vi "ErwKonf_SysLog.vi"(11 "Cluster":T4 {"Lüfter langsam" format="%#_5g"; "Schnell ab:" format="%#_5g"; "FT-IR Kühlung Soll" format="%#_5g"; "FT-IR Kühlung Max" format="%#_5g"; "Stickstoff Befüllzeit" format="%#_5g"; "Befüllintervall" format="%#_5g"; "Kalib.FT-IR" format="%#_5g"; "Offset Ausgang" format="%#_5g"; "Offset FT-IR" format="%#_5g"; "Offset Druck FT-IR" format="%#_5g"; "Dichtheitstest Zeit" format="%#_5g"; "Dichtheitstest Abfall" format="%#_5g"; "Dichtheitstest Umfang" items=["Pumpe / Filter / FT-IR / PNS", "Pumpe / Filter / FT-IR", "Filter / FT-IR", "FT-IR"]; "Offset Umgebung" format="%#_5g"; "Max Taupunkt" format="%#_5g"}) -> (3 "Cluster out":T4 {"Lüfter langsam" format="%#_5g"; "Schnell ab:" format="%#_5g"; "FT-IR Kühlung Soll" format="%#_5g"; "FT-IR Kühlung Max" format="%#_5g"; "Stickstoff Befüllzeit" format="%#_5g"; "Befüllintervall" format="%#_5g"; "Kalib.FT-IR" format="%#_5g"; "Offset Ausgang" format="%#_5g"; "Offset FT-IR" format="%#_5g"; "Offset Druck FT-IR" format="%#_5g"; "Dichtheitstest Zeit" format="%#_5g"; "Dichtheitstest Abfall" format="%#_5g"; "Dichtheitstest Umfang" items=["Pumpe / Filter / FT-IR / PNS", "Pumpe / Filter / FT-IR", "Filter / FT-IR", "FT-IR"]; "Offset Umgebung" format="%#_5g"; "Max Taupunkt" format="%#_5g"})   [LabVIEW 2020, in "Erweiterte Konfig.lvlib"]
uses:
  Erweiterte Konfig.lvlib
  Visualisierungs Elemente/Zahlen-Eingabefeld.ctl
  Visualisierungs Elemente/Auswahlfeld.ctl
  Dichtheitstest Umfang.ctl
  FGV PID Aktionen.ctl
  SysLog/SysLog Interface.ctl
  SysLog/SysLog.lvlib
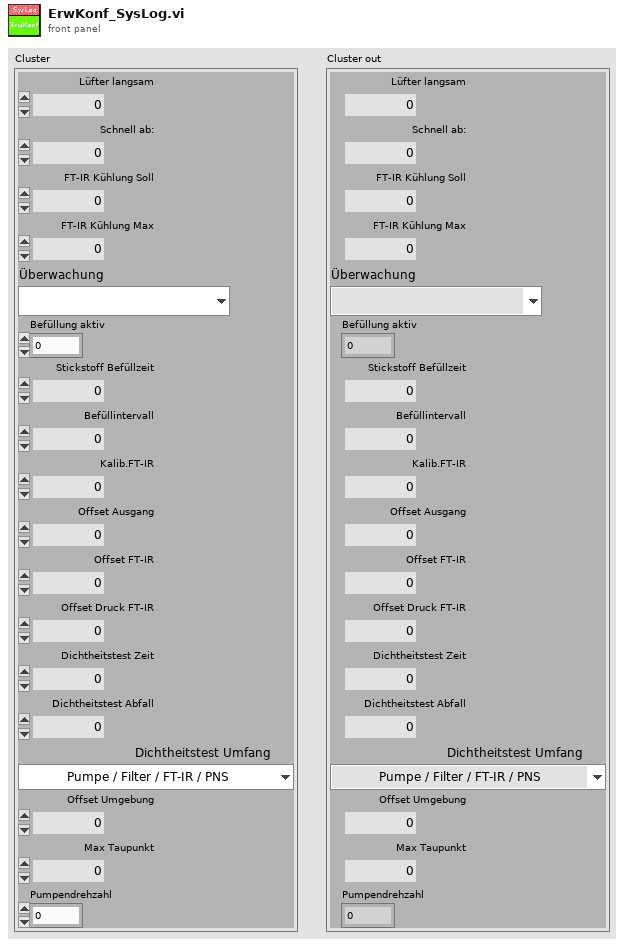
[diagram p1: front panel]
types:
  T1 = typedef "Zahlen-Eingabefeld.ctl" = sgl
  T2 = typedef "Auswahlfeld.ctl" = u16
  T3 = typedef "Erweiterte Konfig.lvlib/Dichtheitstest Umfang.ctl" = u16
  T4 = cluster{"Lüfter langsam":T1, "Schnell ab:":T1, "FT-IR Kühlung Soll":T1, "FT-IR Kühlung Max":T1, "Überwachung":T2, "Befüllung aktiv":u16, "Stickstoff Befüllzeit":T1, "Befüllintervall":T1, "Kalib.FT-IR":T1, "Offset Ausgang":T1, "Offset FT-IR":T1, "Offset Druck FT-IR":T1, "Dichtheitstest Zeit":T1, "Dichtheitstest Abfall":T1, "Dichtheitstest Umfang":T3, "Offset Umgebung":T1, "Max Taupunkt":T1, "Pumpendrehzahl":sgl}
  T5 = typedef "Erweiterte Konfig.lvlib/FGV PID Aktionen.ctl" = enum16{"Lesen", "Schreiben PID", "Schreiben Sonstige", "Dichtheitstest", "Aktionen Dicht.", "Parameter Sensor"}
  T6 = typedef "Erweiterte Konfig.lvlib/Sonstige Parameter.ctl" = cluster{"Lüfter langsam":sgl, "Lüfter schnell":sgl, "FT-IR Kühlung Soll":sgl, "FT-IR Kühlung Max":sgl, "Überwachung":T2, "Befüllung aktiv":T7, "Stickstoff Befüllzeit":sgl, "Befüllintervall":sgl, "Kalibrierwert FT-IR":sgl, "Offset Ausgang":sgl, "Offset FT-IR":sgl, "Offset Druck FT-IR":sgl, "Dichtheitstest Zeit":sgl, "Dichtheitstest Abfall":sgl, "Dichtheitstest Umfang":T3, "Offset Umgebung":sgl, "Max Taupunkt":sgl, "Pumpendrehzahl":sgl}
  T7 = typedef "LogKonfig.lvlib/Auswahlfeld aktiviert-deaktiviert.ctl" = u16
  T8 = typedef "SysLog.lvlib/SysLog Interface.ctl" = cluster{"Fehlermeldung":string, "Erfolgsmeldung":string, "Anzeige":bool, "SysLogIcon":enum16{"OK", "Warnung", "Fehler"}, "intern":bool}
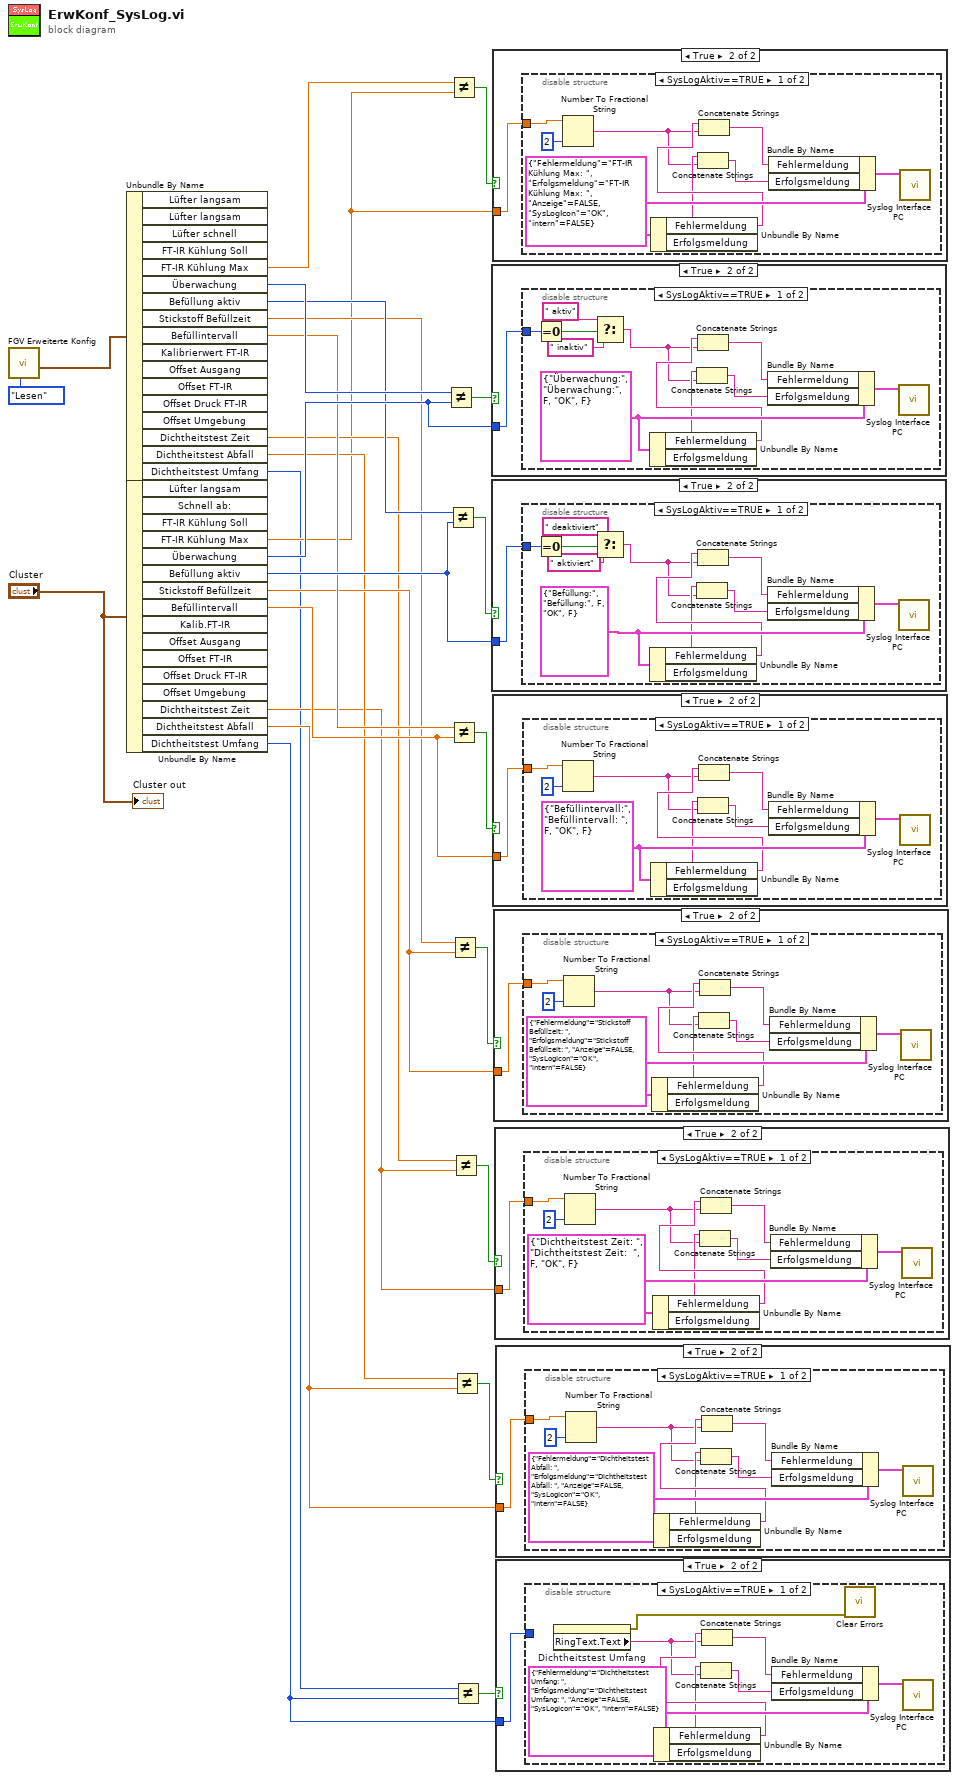
[diagram p0: block diagram]
diagram:
  n1 = call "FGV Erweiterte Konfig.vi"("Aktion"=FGV_PID_Aktionen."Lesen") -> ("Sonstige"=w26:T6)  [unwired: 5 in, 5 out]
  n2 = Unbundle By Name(w26) -> ("FT-IR Kühlung Max"=w5:sgl, "Überwachung"=w24:T2, "Befüllung aktiv"=w21:T7, "Stickstoff Befüllzeit"=w14:sgl, "Befüllintervall"=w17:sgl, "Dichtheitstest Zeit"=w10:sgl, "Dichtheitstest Abfall"=w9:sgl, "Dichtheitstest Umfang"=w3:T3)  [unwired: 9 out]
  n3 = Unbundle By Name("Cluster") -> ("FT-IR Kühlung Max"=w4:T1, "Überwachung"=w22:T2, "Befüllung aktiv"=w19:u16, "Stickstoff Befüllzeit"=w13:T1, "Befüllintervall"=w16:T1, "Dichtheitstest Zeit"=w8:T1, "Dichtheitstest Abfall"=w7:T1, "Dichtheitstest Umfang"=w1:T3)  [unwired: 8 out]
  n4 = Not Equal?(x=w24, y=w22) -> (x != y?=w23:bool)
  n5 = Not Equal?(x=w21, y=w19) -> (x != y?=w20:bool)
  n6 = Not Equal?(x=w5, y=w4) -> (x != y?=w6:bool)
  n7 = Not Equal?(x=w17, y=w16) -> (x != y?=w18:bool)
  n8 = Not Equal?(x=w14, y=w13) -> (x != y?=w15:bool)
  n9 = Not Equal?(x=w10, y=w8) -> (x != y?=w12:bool)
  n10 = Not Equal?(x=w9, y=w7) -> (x != y?=w11:bool)
  n11 = Not Equal?(x=w3, y=w1) -> (x != y?=w2:bool)
  n12 = case shown="True" w23 {
    tunnel: w22 -> [_ w28]
    frame False {
    }
    frame True {
      n13 = disable-structure shown="SysLogAktiv==TRUE" {
        disable-tunnel: w28 -> [w37 _]
        frame condition #0 (active) {
          w39 = T8 {"Fehlermeldung"="Überwachung:", "Erfolgsmeldung"="Überwachung:", "Anzeige"=FALSE, "SysLogIcon"=enum."OK", "intern"=FALSE} ("Cluster (in)")
          n14 = Equal To 0?(x=w37) -> (x = 0?=w38:bool)
          n15 = Select(t=" aktiv", s=w38, f=" inaktiv") -> (s? t:f=w31:string)
          n16 = Unbundle By Name(w39) -> ("Fehlermeldung"=w33:string, "Erfolgsmeldung"=w32:string)
          n17 = Concatenate Strings(w32, w31) -> (w29:string)
          n18 = Concatenate Strings(w33, w31) -> (w30:string)
          n19 = Bundle By Name(cluster=w39, "Fehlermeldung"=w30, "Erfolgsmeldung"=w29) -> (w34:T8)
          n20 = call "Syslog Interface PC.vi"("Cluster (in)"=w34) -> ()  [unwired: 10 in, 1 out]
        }
        frame condition #1 {
        }
      }
    }
  }
  n21 = case shown="True" w20 {
    tunnel: w19 -> [_ w40]
    frame False {
    }
    frame True {
      n22 = disable-structure shown="SysLogAktiv==TRUE" {
        disable-tunnel: w40 -> [w49 _]
        frame condition #0 (active) {
          w51 = T8 {"Fehlermeldung"="Befüllung:", "Erfolgsmeldung"="Befüllung:", "Anzeige"=FALSE, "SysLogIcon"=enum."OK", "intern"=FALSE} ("Cluster (in)")
          n23 = Equal To 0?(x=w49) -> (x = 0?=w50:bool)
          n24 = Select(t=" deaktiviert", s=w50, f=" aktiviert") -> (s? t:f=w43:string)
          n25 = Unbundle By Name(w51) -> ("Fehlermeldung"=w45:string, "Erfolgsmeldung"=w44:string)
          n26 = Concatenate Strings(w44, w43) -> (w41:string)
          n27 = Concatenate Strings(w45, w43) -> (w42:string)
          n28 = Bundle By Name(cluster=w51, "Fehlermeldung"=w42, "Erfolgsmeldung"=w41) -> (w46:T8)
          n29 = call "Syslog Interface PC.vi"("Cluster (in)"=w46) -> ()  [unwired: 10 in, 1 out]
        }
        frame condition #1 {
        }
      }
    }
  }
  n30 = case shown="True" w6 {
    tunnel: w4 -> [_ w52]
    frame False {
    }
    frame True {
      n31 = disable-structure shown="SysLogAktiv==TRUE" {
        disable-tunnel: w52 -> [w55 _]
        frame condition #0 (active) {
          w61 = T8 {"Fehlermeldung"="FT-IR Kühlung Max: ", "Erfolgsmeldung"="FT-IR Kühlung Max: ", "Anzeige"=FALSE, "SysLogIcon"=enum."OK", "intern"=FALSE} ("Cluster (in)")
          n32 = Number To Fractional String(number=w55, precision (6)=i16 2 ("Genauigkeit (6)")) -> (F-format string=w54:string)  [unwired: 2 in]
          n33 = Unbundle By Name(w61) -> ("Fehlermeldung"=w59:string, "Erfolgsmeldung"=w58:string)
          n34 = Concatenate Strings(w58, w54) -> (w56:string)
          n35 = Concatenate Strings(w59, w54) -> (w57:string)
          n36 = Bundle By Name(cluster=w61, "Fehlermeldung"=w57, "Erfolgsmeldung"=w56) -> (w60:T8)
          n37 = call "Syslog Interface PC.vi"("Cluster (in)"=w60) -> ()  [unwired: 10 in, 1 out]
        }
        frame condition #1 {
        }
      }
    }
  }
  n38 = case shown="True" w18 {
    tunnel: w16 -> [_ w62]
    frame False {
    }
    frame True {
      n39 = disable-structure shown="SysLogAktiv==TRUE" {
        disable-tunnel: w62 -> [w65 _]
        frame condition #0 (active) {
          w71 = T8 {"Fehlermeldung"="Befüllintervall:", "Erfolgsmeldung"="Befüllintervall: ", "Anzeige"=FALSE, "SysLogIcon"=enum."OK", "intern"=FALSE} ("Cluster (in)")
          n40 = Number To Fractional String(number=w65, precision (6)=i16 2 ("Genauigkeit (6)")) -> (F-format string=w64:string)  [unwired: 2 in]
          n41 = Unbundle By Name(w71) -> ("Fehlermeldung"=w69:string, "Erfolgsmeldung"=w68:string)
          n42 = Concatenate Strings(w68, w64) -> (w66:string)
          n43 = Concatenate Strings(w69, w64) -> (w67:string)
          n44 = Bundle By Name(cluster=w71, "Fehlermeldung"=w67, "Erfolgsmeldung"=w66) -> (w70:T8)
          n45 = call "Syslog Interface PC.vi"("Cluster (in)"=w70) -> ()  [unwired: 10 in, 1 out]
        }
        frame condition #1 {
        }
      }
    }
  }
  n46 = case shown="True" w15 {
    tunnel: w13 -> [_ w72]
    frame False {
    }
    frame True {
      n47 = disable-structure shown="SysLogAktiv==TRUE" {
        disable-tunnel: w72 -> [w75 _]
        frame condition #0 (active) {
          w81 = T8 {"Fehlermeldung"="Stickstoff Befüllzeit: ", "Erfolgsmeldung"="Stickstoff Befüllzeit: ", "Anzeige"=FALSE, "SysLogIcon"=enum."OK", "intern"=FALSE} ("Cluster (in)")
          n48 = Number To Fractional String(number=w75, precision (6)=i16 2 ("Genauigkeit (6)")) -> (F-format string=w74:string)  [unwired: 2 in]
          n49 = Unbundle By Name(w81) -> ("Fehlermeldung"=w79:string, "Erfolgsmeldung"=w78:string)
          n50 = Concatenate Strings(w78, w74) -> (w76:string)
          n51 = Concatenate Strings(w79, w74) -> (w77:string)
          n52 = Bundle By Name(cluster=w81, "Fehlermeldung"=w77, "Erfolgsmeldung"=w76) -> (w80:T8)
          n53 = call "Syslog Interface PC.vi"("Cluster (in)"=w80) -> ()  [unwired: 10 in, 1 out]
        }
        frame condition #1 {
        }
      }
    }
  }
  n54 = case shown="True" w12 {
    tunnel: w8 -> [_ w82]
    frame False {
    }
    frame True {
      n55 = disable-structure shown="SysLogAktiv==TRUE" {
        disable-tunnel: w82 -> [w85 _]
        frame condition #0 (active) {
          w91 = T8 {"Fehlermeldung"="Dichtheitstest Zeit: ", "Erfolgsmeldung"="Dichtheitstest Zeit:  ", "Anzeige"=FALSE, "SysLogIcon"=enum."OK", "intern"=FALSE} ("Cluster (in)")
          n56 = Number To Fractional String(number=w85, precision (6)=i16 2 ("Genauigkeit (6)")) -> (F-format string=w84:string)  [unwired: 2 in]
          n57 = Unbundle By Name(w91) -> ("Fehlermeldung"=w89:string, "Erfolgsmeldung"=w88:string)
          n58 = Concatenate Strings(w88, w84) -> (w86:string)
          n59 = Concatenate Strings(w89, w84) -> (w87:string)
          n60 = Bundle By Name(cluster=w91, "Fehlermeldung"=w87, "Erfolgsmeldung"=w86) -> (w90:T8)
          n61 = call "Syslog Interface PC.vi"("Cluster (in)"=w90) -> ()  [unwired: 10 in, 1 out]
        }
        frame condition #1 {
        }
      }
    }
  }
  n62 = case shown="True" w11 {
    tunnel: w7 -> [_ w92]
    frame False {
    }
    frame True {
      n63 = disable-structure shown="SysLogAktiv==TRUE" {
        disable-tunnel: w92 -> [w95 _]
        frame condition #0 (active) {
          w101 = T8 {"Fehlermeldung"="Dichtheitstest Abfall: ", "Erfolgsmeldung"="Dichtheitstest Abfall: ", "Anzeige"=FALSE, "SysLogIcon"=enum."OK", "intern"=FALSE} ("Cluster (in)")
          n64 = Number To Fractional String(number=w95, precision (6)=i16 2 ("Genauigkeit (6)")) -> (F-format string=w94:string)  [unwired: 2 in]
          n65 = Unbundle By Name(w101) -> ("Fehlermeldung"=w99:string, "Erfolgsmeldung"=w98:string)
          n66 = Concatenate Strings(w98, w94) -> (w96:string)
          n67 = Concatenate Strings(w99, w94) -> (w97:string)
          n68 = Bundle By Name(cluster=w101, "Fehlermeldung"=w97, "Erfolgsmeldung"=w96) -> (w100:T8)
          n69 = call "Syslog Interface PC.vi"("Cluster (in)"=w100) -> ()  [unwired: 10 in, 1 out]
        }
        frame condition #1 {
        }
      }
    }
  }
  n70 = case shown="True" w2 {
    tunnel: w1 -> [_ w102]
    frame False {
    }
    frame True {
      n71 = disable-structure shown="SysLogAktiv==TRUE" {
        disable-tunnel: w102 -> [_ _]
        frame condition #0 (active) {
          w110 = T8 {"Fehlermeldung"="Dichtheitstest Umfang: ", "Erfolgsmeldung"="Dichtheitstest Umfang: ", "Anzeige"=FALSE, "SysLogIcon"=enum."OK", "intern"=FALSE} ("Cluster (in)")
          n72 = property on="Dichtheitstest Umfang" class="Ring (strikt)"() -> (error out=w103:errorcluster, "RingText.Text"=w104:string)  [unwired: 2 in, 1 out]
          n73 = Unbundle By Name(w110) -> ("Fehlermeldung"=w108:string, "Erfolgsmeldung"=w107:string)
          n74 = Concatenate Strings(w107, w104) -> (w105:string)
          n75 = Concatenate Strings(w108, w104) -> (w106:string)
          n76 = Bundle By Name(cluster=w110, "Fehlermeldung"=w106, "Erfolgsmeldung"=w105) -> (w109:T8)
          n77 = call <vilib>:"Clear Errors.vi"("error in (no error)"=w103) -> ()  [unwired: 5 in, 2 out]
          n78 = call "Syslog Interface PC.vi"("Cluster (in)"=w109) -> ()  [unwired: 10 in, 1 out]
        }
        frame condition #1 {
        }
      }
    }
  }
  "Cluster out" <- "Cluster"
